vi "Import File - Main XML.vi"(6 "Root Node":refnum<k24>, 8 "error in (no error)":errorcluster) -> (0 "error out":errorcluster, 5 "Import/Export Data - Main":T1)   [LabVIEW 2016, in "UDP-Custom-Device System Explorer.lvlib"]
uses:
  UDP-Custom-Device System Explorer.lvlib
  System.Xml
  Types/XML - New/ImpExp - Main Data.ctl
  <vilib>/NI Veristand/Custom Device API/Custom Device Item Info.ctl
  <vilib>/NI VeriStand/Custom Device API/Custom Device API.lvlib
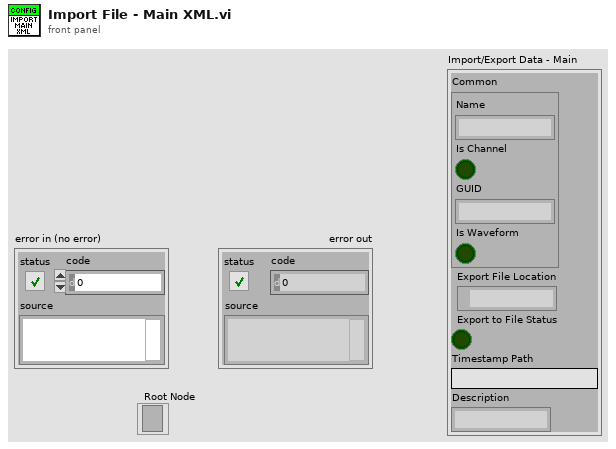
[diagram p1: front panel]
types:
  T1 = typedef "UDP-Custom-Device System Explorer.lvlib/ImpExp - Main Data.ctl" = cluster{"Common":T2, "Export File Location":path, "Export to File Status":bool, "Timestamp Path":string, "Description":string}
  T2 = typedef "Custom Device API.lvlib/Custom Device Item Info.ctl" = cluster{"Name":string, "Is Channel":bool, "GUID":string, "Is Waveform":bool}
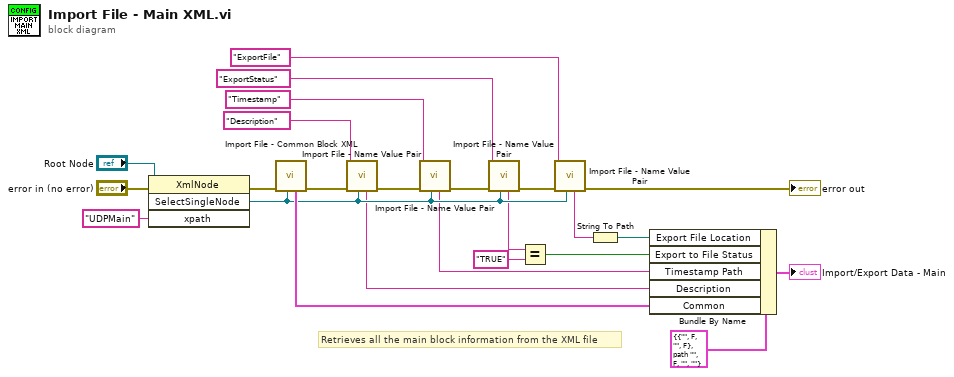
[diagram p0: block diagram]
diagram:
  # "Retrieves all the main block information from the XML file"
  n1 = invoke class="XmlNode" method="SelectSingleNode"(reference="Root Node", error in="error in (no error)", "xpath"="UDPMain") -> (error out=w21:errorcluster, "SelectSingleNode"=w11:refnum<k24>)  [unwired: 1 in, 2 out]
  n2 = call "Import File - Common Block XML.vi"("Root Node"=w11, "error in (no error)"=w21) -> ("error out"=w17:errorcluster, "Common"=w19:T2)  [unwired: 8 in]
  n3 = call "Import File - Name Value Pair.vi"("Root Node"=w11, "error in (no error)"=w17, "Node Name"="Description") -> ("error out"=w16:errorcluster, "Value"=w7:string)  [unwired: 7 in]
  n4 = call "Import File - Name Value Pair.vi"("Root Node"=w11, "error in (no error)"=w16, "Node Name"="Timestamp") -> ("error out"=w15:errorcluster, "Value"=w6:string)  [unwired: 7 in]
  n5 = call "Import File - Name Value Pair.vi"("Root Node"=w11, "error in (no error)"=w15, "Node Name"="ExportStatus") -> ("error out"=w14:errorcluster, "Value"=w4:string)  [unwired: 7 in]
  n6 = Equal?(x=w4, y="TRUE") -> (x = y?=w3:bool)
  n7 = call "Import File - Name Value Pair.vi"("Root Node"=w11, "error in (no error)"=w14, "Node Name"="ExportFile") -> ("error out"=→"error out":errorcluster, "Value"=w2:string)  [unwired: 7 in]
  n8 = String To Path(string=w2) -> (path=w1:path)
  n9 = Bundle By Name(cluster=T1 {"Common"={"Name"="", "Is Channel"=FALSE, "GUID"="", "Is Waveform"=FALSE}, "Export File Location"=path "", "Export to File Status"=FALSE, "Timestamp Path"="", "Description"=""} ("Import/Export Data - Main"), "Export File Location"=w1, "Export to File Status"=w3, "Timestamp Path"=w6, "Description"=w7, "Common"=w19) -> (→"Import/Export Data - Main":T1)
